vi "FT10_Fornax Enable DFT.vi"(11 "Message Handling Cluster in":T1) -> (3 "Message Handling Cluster out":T1)   [LabVIEW 2015]
uses:
  Controls/Control_Message Handling Cluster.ctl
  Controls/Control_M4X Connection.ctl
  Controls/Control_PXI-7854R FPGA Reference.ctl
  Controls/Control_Config Cluster.ctl
  Controls/Control_Config Unitherm Port.ctl
  Controls/Control_Config Simulate Values.ctl
  Controls/Control_Log Queue.ctl
  Controls/Control_Log Cluster.ctl
  Controls/Control_Log Time.ctl
  Controls/Control_Log Waveform Cluster.ctl
  Controls/Control_Log Analysis Cluster.ctl
  Controls/Control_Log Flag.ctl
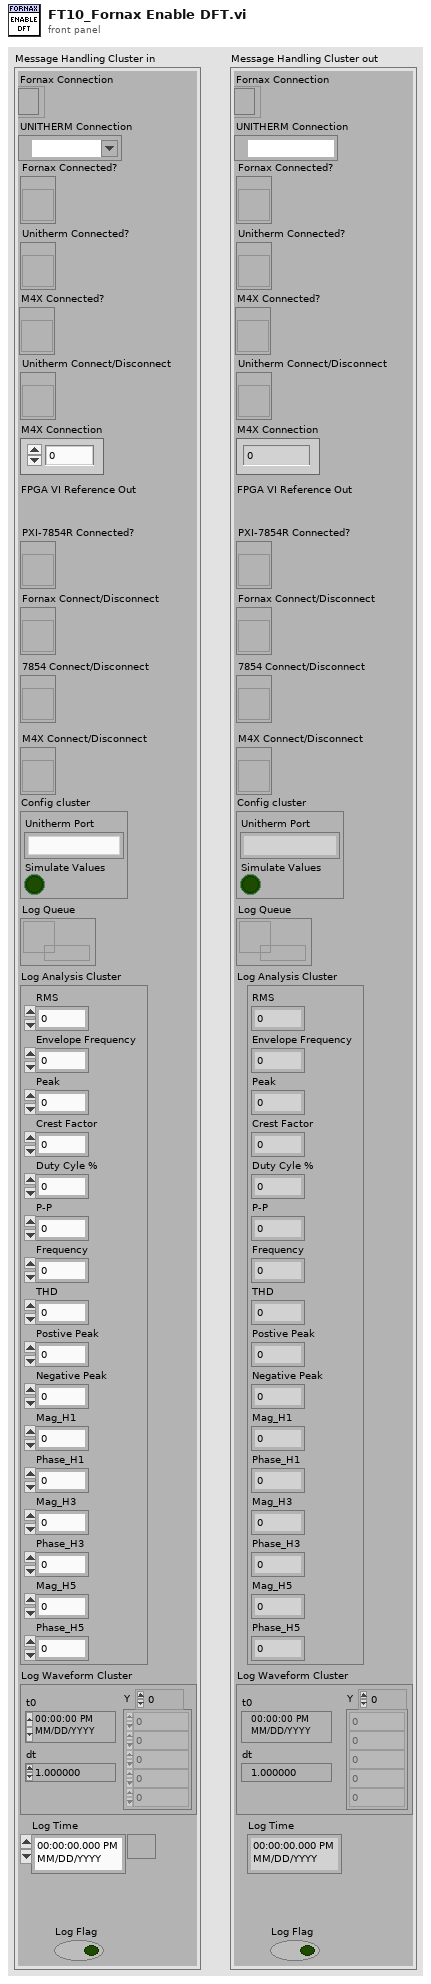
[diagram p1: front panel]
types:
  T1 = typedef "Control_Message Handling Cluster.ctl" = cluster{"Fornax Connected?":refnum<vi>, "Unitherm Connected?":refnum<vi>, "M4X Connected?":refnum<vi>, "Unitherm Connect/Disconnect":refnum<vi>, "Fornax Connection":refnum<k5>, "UNITHERM Connection":refnum<visa-resource-name>, "M4X Connection":T2, "PXI-7854R FPGA Reference":T3, "PXI-7854R Connected?":refnum<vi>, "Fornax Connect/Disconnect":refnum<vi>, "7854 Connect/Disconnect":refnum<vi>, "M4X Connect/Disconnect":refnum<vi>, "Config Cluster":T4, "Log Queue":T7, "Log Analysis Cluster":T8, "Log Waveform Cluster":T9, "Log Time":T10, "Log Flag":T11}
  T2 = typedef "Control_M4X Connection.ctl" = u32
  T3 = typedef "Control_PXI-7854R FPGA Reference.ctl" = refnum<k20>
  T4 = typedef "Control_Config Cluster.ctl" = cluster{"Unitherm Port":T5, "Simulate Values":T6}
  T5 = typedef "Control_Config Unitherm Port.ctl" = string
  T6 = typedef "Control_Config Simulate Values.ctl" = bool
  T7 = typedef "Control_Log Queue.ctl" = refnum<queue>
  T8 = typedef "Control_Log Analysis Cluster.ctl" = cluster{"RMS":dbl, "Envelope Frequency":dbl, "Peak":dbl, "Crest Factor":dbl, "Duty Cyle %":dbl, "P-P":dbl, "Frequency":dbl, "THD":dbl, "Postive Peak":dbl, "Negative Peak":dbl, "Mag_H1":dbl, "Phase_H1":dbl, "Mag_H3":dbl, "Phase_H3":dbl, "Mag_H5":dbl, "Phase_H5":dbl}
  T9 = typedef "Control_Log Waveform Cluster.ctl" = waveform(dbl)
  T10 = typedef "Control_Log Time.ctl" = timestamp
  T11 = typedef "Control_Log Flag.ctl" = bool
  T12 = enum16{"EXTERNAL_COMM_COMMAND_INVALID", "EXTERNAL_COMM_COMMAND_PAIR_VLEX", "EXTERNAL_COMM_COMMAND_PAIR_FORNAX", "EXTERNAL_COMM_COMMAND_PAIR_INTEGRATION_TESTOR", "EXTERNAL_COMM_COMMAND_ENABLE_DFA", "EXTERNAL_COMM_COMMAND_ENABLE_DFT", "EXTERNAL_COMM_COMMAND_ENABLE_VIPER", "EXTERNAL_COMM_COMMAND_AUTO_ETHERNET_ON", "EXTERNAL_COMM_COMMAND_AUTO_ETHERNET_OFF", "EXTERNAL_COMM_COMMAND_STREAM_RFDATA_ON", "EXTERNAL_COMM_COMMAND_STREAM_RFDATA_OFF", "EXTERNAL_COMM_COMMAND_STREAM_ISOFIRM_ON", "EXTERNAL_COMM_COMMAND_STREAM_ISOFIRM_OFF", "EXTERNAL_COMM_COMMAND_STREAM_RFID_ON", "EXTERNAL_COMM_COMMAND_STREAM_RFID_OFF", "EXTERNAL_COMM_COMMAND_AUTO_ETHERNET_ONCE"}
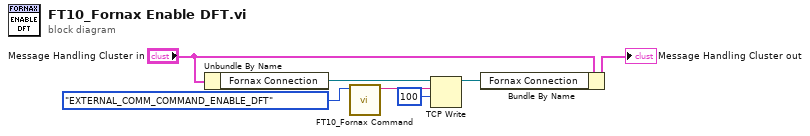
[diagram p0: block diagram]
diagram:
  n1 = Unbundle By Name("Message Handling Cluster in") -> ("Fornax Connection"=w4:refnum<k5>)
  n2 = call "FT10_Fornax Command.vi"("ExternalCommCommand"=T12."EXTERNAL_COMM_COMMAND_ENABLE_DFT") -> ("JSON Message"=w7:string)  [unwired: 10 in]
  n3 = TCP Write(connection ID=w4, data in=w7, 9:100 ("timeout ms (25000)")) -> (connection ID out=w5:refnum<k5>)  [unwired: 1 in, 2 out]
  n4 = Bundle By Name(cluster="Message Handling Cluster in", "Fornax Connection"=w5) -> (→"Message Handling Cluster out":T1)
